vi "JYMirrorMove.vi"(7 "UniqueID":string, 8 "error in (no error)":errorcluster, 9 "Mirror Position":u16(ring) items=["Front", "Side"], 10 "Mirror Number":u16(ring) items=["Entrance", "Exit"], 11 "RefNum In":refnum<k7>) -> (0 "error out":errorcluster, 3 "MonoRefNum Out":refnum<k7>)   [LabVIEW 2009]
doc: "JYMirrorMove.vi\n\nMove the mirror on a mono. There are 2 modes of operation; local or\nremote. The local mode allows the mirror number and position to be set\nvia the front panel controls. Note that the front panel will not be displayed in local mode. The remole mode allows the values to be supplied\nprogrammatically. \n\nEither a UniqueID or a valid refnum can be supplied to the VI. If the UniqueID is supplied, the InitMono VI will be executed and a new refnum will be generated. It is up to the user to manage the automation refnums.\n\nInputs\nMonoRefNum - LabView automation refnum. This is an existing valid automation refnum\n\nMono UniqueID - The Unique ID of the mono.\n\nExt Mirror Number - Must be supplied for remote operation. Not required\n for front panel operation\n\nExt Mirror Position - Must be supplied for remote operation. Not required\n for front panel operation\n\nInput Error Cluster -\n\n----------------------------------------------------------\nOutputs\n\nAutomation refnum - If a valid automation refnum is supplied as an input, this will be supplied at the output. If a unique ID was supplied, the output refnum will be a newly generated refnum.\n \nOutput Error Cluster"
panel:
  out "UseUniqueID":bool
  in  "Input Select":bool
  # "Local / Front Panel Mode"
  # "Remote / Program Mode"
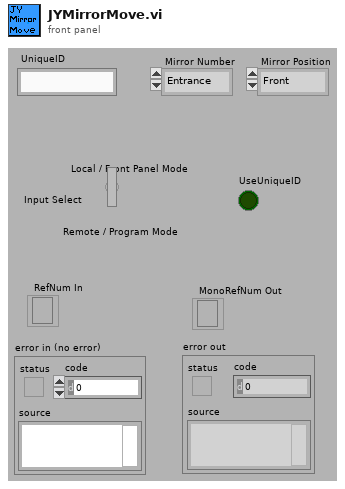
[diagram p1: front panel]
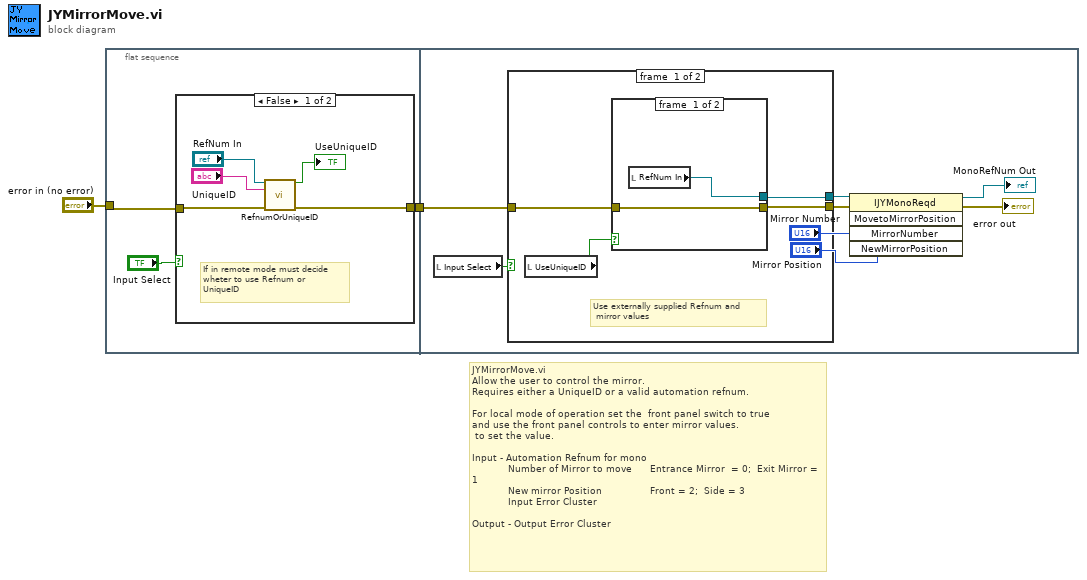
[diagram p0: block diagram]
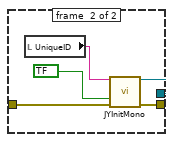
[diagram p3: hidden frame]
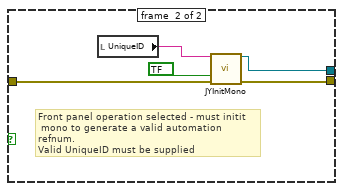
[diagram p4: hidden frame]
diagram:
  # "JYMirrorMove.vi\nAllow the user to control the mirror.\nRequires either a UniqueID or a valid automation refnum.  \n \nFor local mode of operation set the  front panel switch to true\nand use the front panel controls to enter mirror values.\n to set the value.\n\nInput - Automation Refnum for mono\n            Number of Mirror to move      Entrance Mirror  = 0;  Exit Mirror = 1\n            New mirror Position                Front = 2;  Side = 3\n            Input Error Cluster\n\nOutput - Output Error Cluster"
  n1 = flat-sequence {
    tunnel: "error in (no error)" -> [w4]
    tunnel: [w3] -> w1
    tunnel: w1 -> [w14]
    frame #0 {
      n2 = case shown="False" "Input Select" {
        tunnel: w4 -> [w8 w11]
        tunnel: [w7 w11] -> w3
        frame #0 {
          # "If in remote mode must decide\nwheter to use Refnum or \nUniqueID"
          n3 = call "RefnumOrUniqueID.vi"("Refnum IN"="RefNum In", "String in"="UniqueID", "error in (no error)"=w8) -> ("UseUniqueID"=→"UseUniqueID":bool, "error out"=w7:errorcluster)  [unwired: 11 out]
        }
        frame #1 {
        }
      }
    }
    frame #1 {
      n4 = local read "Input Select"() -> (w15:bool)
      n5 = case shown="True" w15 {
        tunnel: [w23 w34] -> w16
        tunnel: [w20 w33] -> w17
        tunnel: w14 -> [w22 w31]
        frame #0 {
          # "Use externally supplied Refnum and\n mirror values"
          n6 = local read "UseUniqueID"() -> (w21:bool)
          n7 = case shown="True" w21 {
            tunnel: [w25 w28] -> w20
            tunnel: [w24 w27] -> w23
            tunnel: w22 -> [w24 w26]
            frame #0 {
              n8 = local read "RefNum In"() -> (w25:refnum<k7>)
            }
            frame #1 {
              n9 = local read "UniqueID"() -> (w30:string)
              n10 = call "JYInitMono.vi"("Unique ID"=w30, "Force Init"=bool ?, "error in (no error)"=w26) -> ("Mono RefNum out"=w28:refnum<k7>, "error out"=w27:errorcluster)  [unwired: 1 in, 10 out]
            }
          }
        }
        frame #1 {
          # "Front panel operation selected - must initit\n mono to generate a valid automation refnum.\nValid UniqueID must be supplied"
          n11 = local read "UniqueID"() -> (w32:string)
          n12 = call "JYInitMono.vi"("Unique ID"=w32, "Force Init"=bool ?, "error in (no error)"=w31) -> ("Mono RefNum out"=w33:refnum<k7>, "error out"=w34:errorcluster)  [unwired: 1 in, 10 out]
        }
      }
      n13 = invoke class="IJYMonoReqd" method="MovetoMirrorPosition"(reference=w17, error in=w16, "MirrorNumber"="Mirror Number", "NewMirrorPosition"="Mirror Position") -> (reference out=→"MonoRefNum Out":refnum<k7>, error out=→"error out":errorcluster)  [unwired: 1 in, 3 out]
    }
  }
